vi "Send Cmd Save Config.vi"(8 "error in (no error)":errorcluster, 11 "Configuration Window in":refnum<class "Configuration Window.lvclass">) -> (0 "error out":errorcluster, 3 "Configuration Window out":refnum<class "Configuration Window.lvclass">)   [LabVIEW 2018, in "Configuration Window.lvlib" / "Configuration Window.lvclass"]
uses:
  Configuration Window.lvclass
  C:/Program Files (x86)/National Instruments/LabVIEW 2018/vi.lib/ActorFramework/Actor/Actor.lvclass
  Main Panel/LF2R IDE/LF2R IDE Cmd.ctl
  <vilib>/ActorFramework/Actor/Actor.lvclass/Actor.ctl
  Main Panel/LF2R IDE Messages/LF2R IDE Cmd Msg/LF2R IDE Cmd Msg.lvclass/LF2R IDE Cmd Msg.ctl
  <vilib>/ActorFramework/Message Enqueuer/Message Enqueuer.lvclass/Message Enqueuer.ctl
  <vilib>/ActorFramework/Message Enqueuer/Enqueue.vi
  Main Panel/LF2R IDE Messages/LF2R IDE Cmd Msg/LF2R IDE Cmd Msg.lvclass
  C:/Program Files (x86)/National Instruments/LabVIEW 2018/vi.lib/ActorFramework/Message/Message.lvclass
  <vilib>/ActorFramework/Message Priority Queue/Priority Enqueue.vi
  <vilib>/ActorFramework/Actor/Actor.lvclass
  Main Panel/LF2R IDE/Main Panel.lvclass
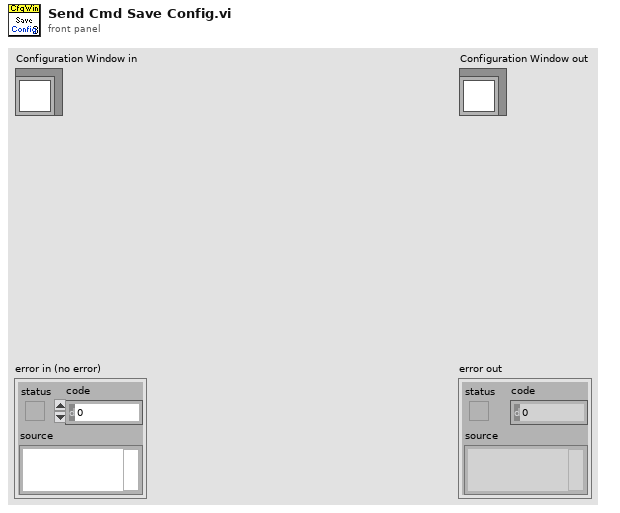
[diagram p1: front panel]
types:
  T1 = typedef "Main Panel.lvlib/Main Panel.lvclass/LF2R IDE Cmd.ctl" = enum16{"Save Data File", "Write Configuration", "Save Configuration", "Update Frame Image"}
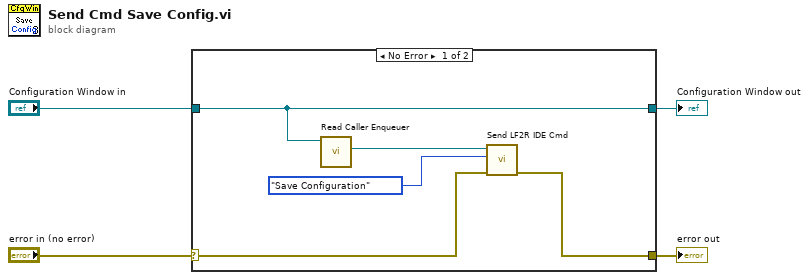
[diagram p0: block diagram]
diagram:
  n1 = case shown="No Error" "error in (no error)" {
    selector: "error in (no error)" -> [w6 w11]
    tunnel: [w5 w11] -> w3
    tunnel: [w9 w10] -> w1
    tunnel: "Configuration Window in" -> [w9 w10]
    frame No Error {
      n2 = call <vilib>:"Read Caller Enqueuer.vi"("Actor"=w9) -> ("Caller Enqueuer"=w8:refnum<class "Message Enqueuer.lvclass">)  [unwired: 10 in]
      n3 = call "Send LF2R IDE Cmd.vi"("error in (no error)"=w6, "CMD"=LF2R_IDE_Cmd."Save Configuration", "Message Enqueuer"=w8) -> ("error out"=w5:errorcluster)  [unwired: 7 in, 1 out]
    }
    frame Error {
    }
  }
  "error out" <- w3
  "Configuration Window out" <- w1
